vi "Shell.vi"(8 "Error In":errorcluster, 11 "Channel In":refnum<class "Channel.lvclass">) -> (0 "Error Out":errorcluster, 3 "Channel Out":refnum<class "Channel.lvclass">)   [LabVIEW 2021, in "Field_RnD_Services_LIBSSH2_Toolkit.lvlib" / "Channel.lvclass"]
doc: "Creates a Shell channel for bidirectional communication with a STDIN, STDOUT, and STDERR streams."
uses:
  Channel.lvclass
  Channel.lvclass/Channel.ctl
  Session/Session.lvclass
  Field_RnD_Services_LIBSSH2_Toolkit.lvlib
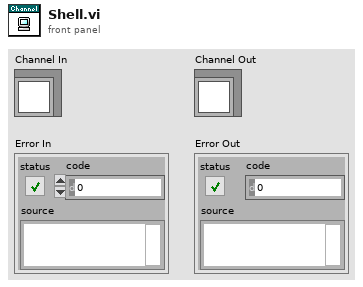
[diagram p1: front panel]
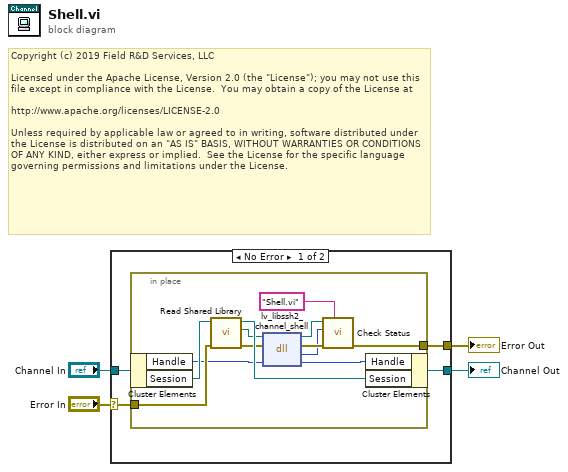
[diagram p0: block diagram]
diagram:
  # "Copyright (c) 2019 Field R&D Services, LLC\n\nLicensed under the Apache License, Version 2.0 (the \"License\"); you may not use this file except in compliance with the License.  You may obtain a copy of the License at\n\nhttp://www.apache.org/licenses/LICENSE-2.0\n\nUnless required by applicable law or agreed to in writing, software distributed under the License is distributed on an \"AS IS\" BASIS, WITHOUT WARRANTIES OR CONDITIONS OF ANY KIND, either express or implied.  See the License for the specific language governing permissions and limitations under the License."
  n1 = case shown="No Error" "Error In" {
    selector: "Error In" -> [w6 w22]
    tunnel: [w5 w22] -> w3
    tunnel: "Channel In" -> [w8 w21]
    tunnel: [w7 w21] -> w1
    frame No Error {
      n2 = in-place {
        in-place-border: w6 -> [w16]
        in-place-border: [w12] -> w5
        n3 = in-place-cluster #1(w8) -> ("Handle"=w11:u64, "Session"=w20:refnum<class "Session.lvclass">)
        n4 = call "Read Shared Library.vi"("Error In"=w16, "Session In"=w20) -> ("Erorr Out"=w17:errorcluster, "libssh2lv Shared Library"=w18:path, "Session Out"=w19:refnum<class "Session.lvclass">)  [unwired: 7 in]
        n5 = dll-call lib="libssh2lv.*" fn="lv_libssh2_channel_shell"(path in=w18, error in=w17, "handle"=w11) -> (path out=w14:path, error out=w15:errorcluster, "status"=w13:i32, "handle"=w10:u64)  [unwired: 1 in]
        n6 = call "Check Status.vi"("Source (\"\")"="Shell.vi" ("Source (\"\")"), "Error In"=w15, "Status"=w13, "libssh2lv Shared Library In"=w14) -> ("Error Out"=w12:errorcluster)  [unwired: 6 in, 1 out]
        n7 = in-place-cluster #1("Handle"=w10, "Session"=w19) -> (w7:refnum<class "Channel.lvclass">)
      }
    }
    frame Error {
    }
  }
  "Error Out" <- w3
  "Channel Out" <- w1
